vi "Main.vi"() -> ()   [LabVIEW 2015]
uses:
  Type defs/System states.ctl
  Type defs/TS UI Data.ctl
  C:/C-BOX_DoIP/Utilities/dotNET/C-BOX_DoIP/C_Box.NET_Utilities.dll
  C-BOX_DoIP/Utilities/dotNET/C-BOX_DoIP/C_Box.NET_Utilities.dll
  Type defs/Nest cluster.ctl
panel:
  in  "Nest cluster":T1={"Main messages"="", "Datamatrix"="", "Barcode"="", "Battery Voltage"="", "Scanned Hardware PN"="", "Scanned Spare PN"="", "Scanned Hardware Version"="", "Scanner Software Version"="", "Scanned Serial ID"="", "Scanned FAZIT"="", "ITAC Hardware PN"="", "ITAC Spare PN"="", "ITAC Hardware Version"="", "ITAC Software Version"="", "ITAC Serial ID"="", "ITAC FAZIT"="", "DoIP Hardware PN"="", "DoIP Spare PN"="", "DoIP Hardware Version\nDoIP Software Version"="", "DoIP Software Version"="", "DoIP Serial ID"="", "DoIP FAZIT"="", "Elapsed time"="0 seg", "Progress slider"=0.0, "System errors"=""} {"Progress slider" scale=0.1..100.0}
  in  "TestStand UI ListBar":refnum<k7>(container)
  in  "TestStand UI SequenceView":refnum<k7>(container)
  in  "Trace Enabled":refnum<k7>(container)
  in  "Sequence File Label":refnum<k7>(container) caption="Secuencia:"
  in  "Stop Button":refnum<k7>(container)
  in  "Start Button":refnum<k7>(container)
  in  "Exit Button":refnum<k7>(container)
  in  "error in (no error)":errorcluster
  in  "Reset Button":bool
  in  "Yield:":string="-"
  in  "Bad:":string="-" caption="Malas:"
  in  "Good:":string="-" caption="Buenas:"
  in  "Total:":string="-"
  in  "Info Button":bool
  in  "Settings Button":bool
  in  "TestStand UI ExecutionView Manager":refnum<k7>(container)
  in  "TestStand UI SequenceFileView Manager":refnum<k7>(container)
  in  "TestStand UI Application Manager":refnum<k7>(container)
  in  "Main message":string
  # "SCANNED DATA"
  # "ITAC DATA"
  # "DoIP DATA"
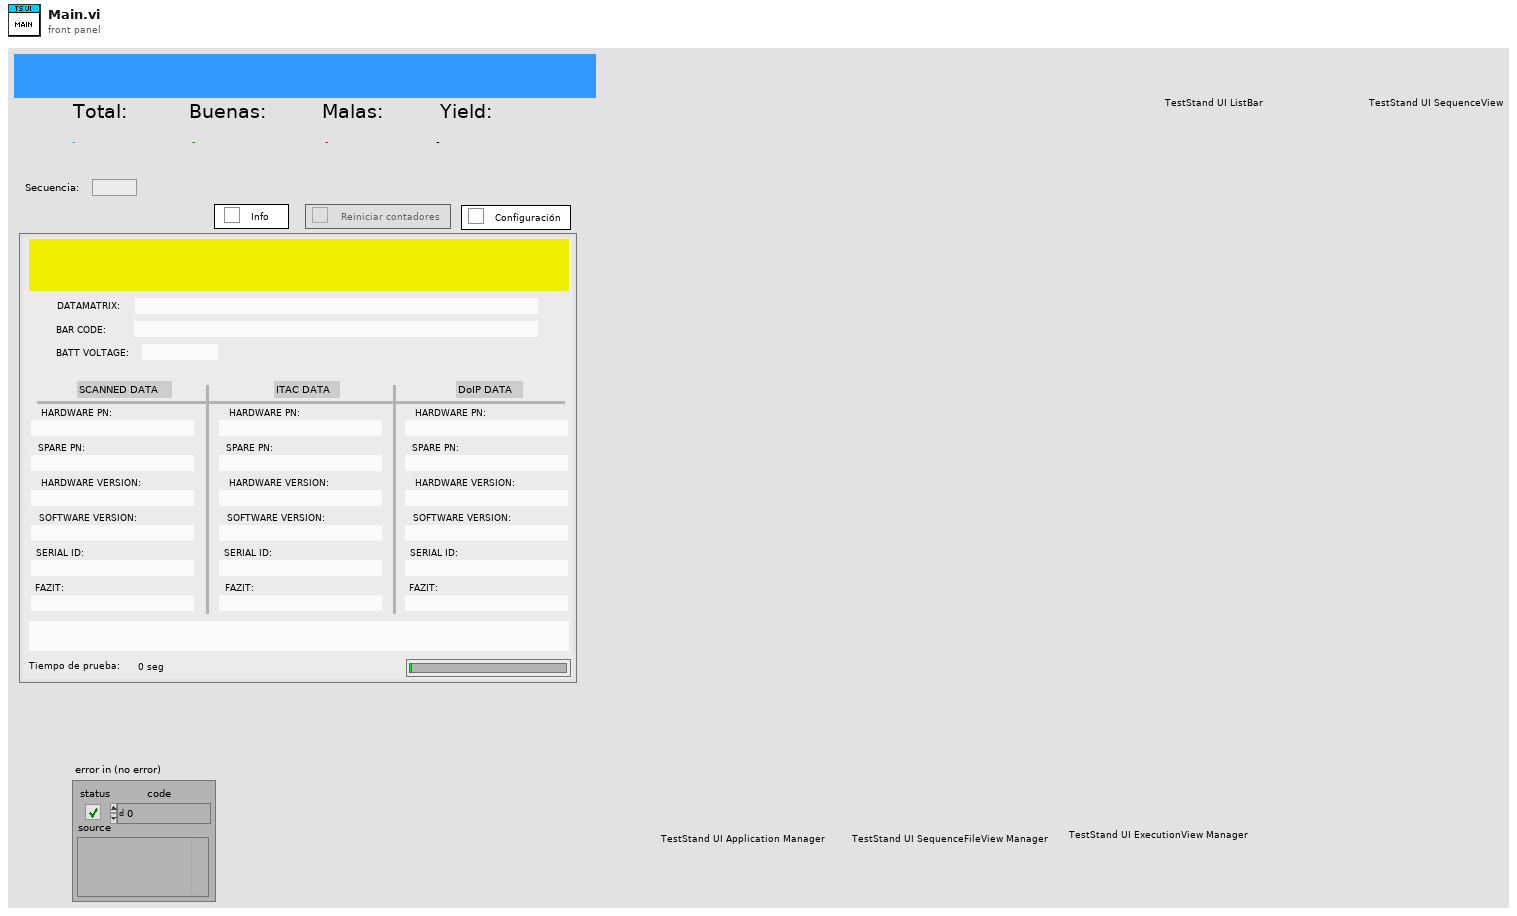
[diagram p1: front panel]
types:
  T1 = typedef "Nest cluster.ctl" = cluster{"Main messages":string, "Datamatrix":string, "Barcode":string, "Battery Voltage":string, "Scanned Hardware PN":string, "Scanned Spare PN":string, "Scanned Hardware Version":string, "Scanner Software Version":string, "Scanned Serial ID":string, "Scanned FAZIT":string, "ITAC Hardware PN":string, "ITAC Spare PN":string, "ITAC Hardware Version":string, "ITAC Software Version":string, "ITAC Serial ID":string, "ITAC FAZIT":string, "DoIP Hardware PN":string, "DoIP Spare PN":string, "DoIP Hardware Version\nDoIP Software Version":string, "DoIP Software Version":string, "DoIP Serial ID":string, "DoIP FAZIT":string, "Elapsed time":string, "Progress slider":dbl, "System errors":string}
  T2 = typedef "TS UI Data.ctl" = cluster{"Other references":cluster{"event callback refnum":refnum<k27>, "Quit Application Event":refnum<user-event>, "Change nest message bgcolor Event":refnum<user-event>, "event registration refnum":refnum<event-registration>, "Top Level VI":refnum<vi>, "TS.IEngine":refnum<k7>, "Nest Cluster":refnum<vi>}, "Manager controls":cluster{"TSUI.IApplicationMgr":refnum<k7>, "TSUI.ISequenceFileViewMgr":refnum<k7>, "TSUI.IExecutionViewMgr":refnum<k7>}, "Visible controls":cluster{"Start Button":refnum<k7>, "Stop Button":refnum<k7>, "Info Button":refnum<vi>, "Settings Button":refnum<vi>, "Reset Counters Button":refnum<vi>, "Exit Button":refnum<k7>, "Main message":refnum<vi>, "Part number":refnum<vi>, "Total counter":refnum<vi>, "Good counter":refnum<vi>, "Bad counter":refnum<vi>, "Yield":refnum<vi>, "Sequence File Label":refnum<k7>, "Trace Enabled":refnum<k7>, "Sequence View":refnum<k7>, "Sequence Execution":refnum<k7>}}
  T3 = typedef "System states.ctl" = enum16{"Init", "Configure connections", "Register callbacks", "Start application", "Event handler", "Error handler", "Shutdown"}
  T4 = enum32{"invalid app kind", "Development System", "Run Time System", "Student Edition", "Embedded LabVIEW", "Evaluation", "Custom"}
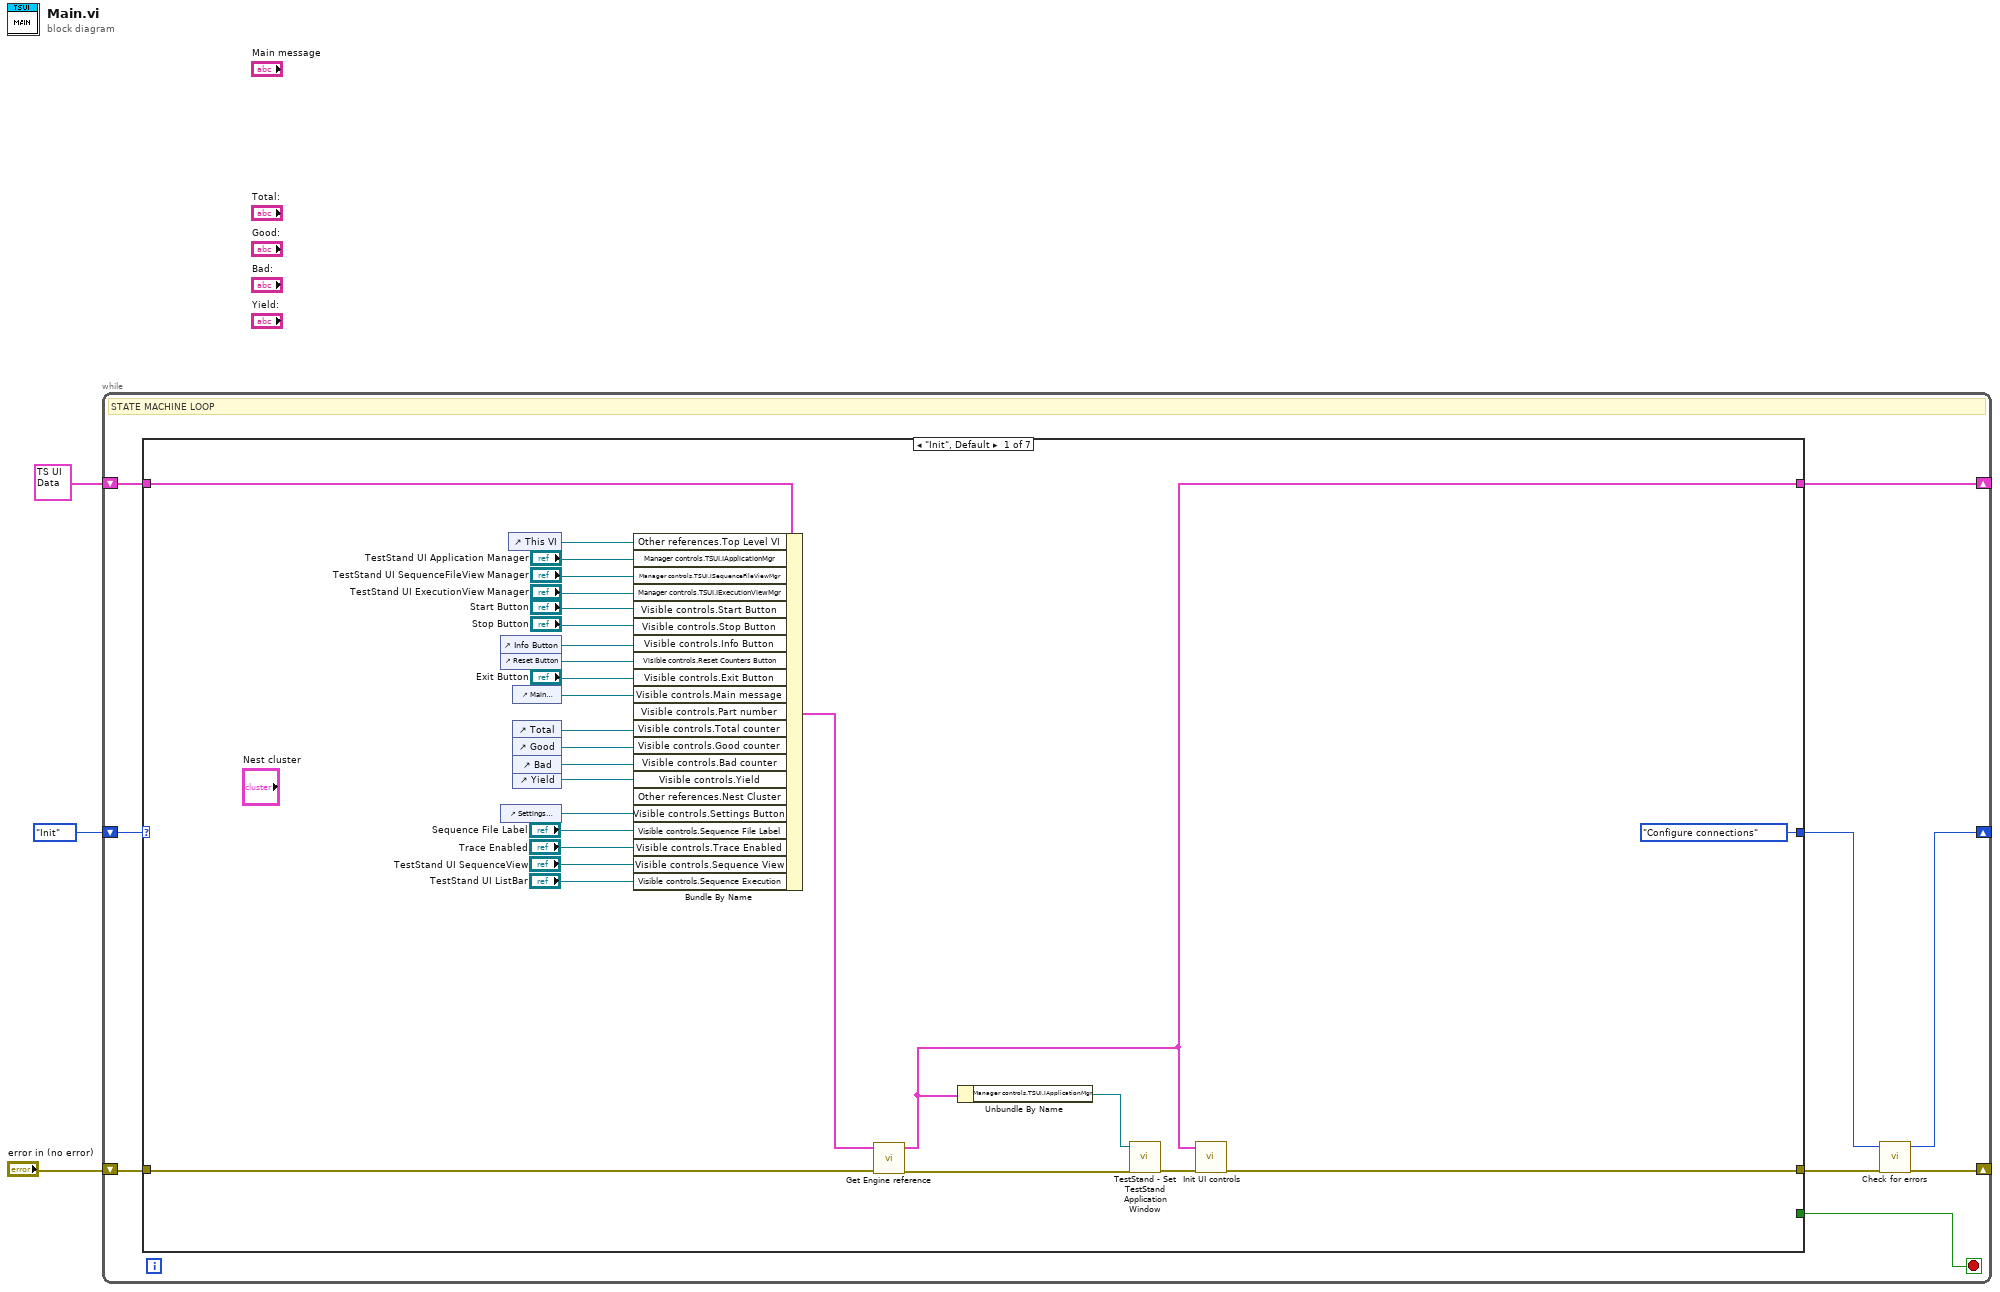
[diagram p0: block diagram]
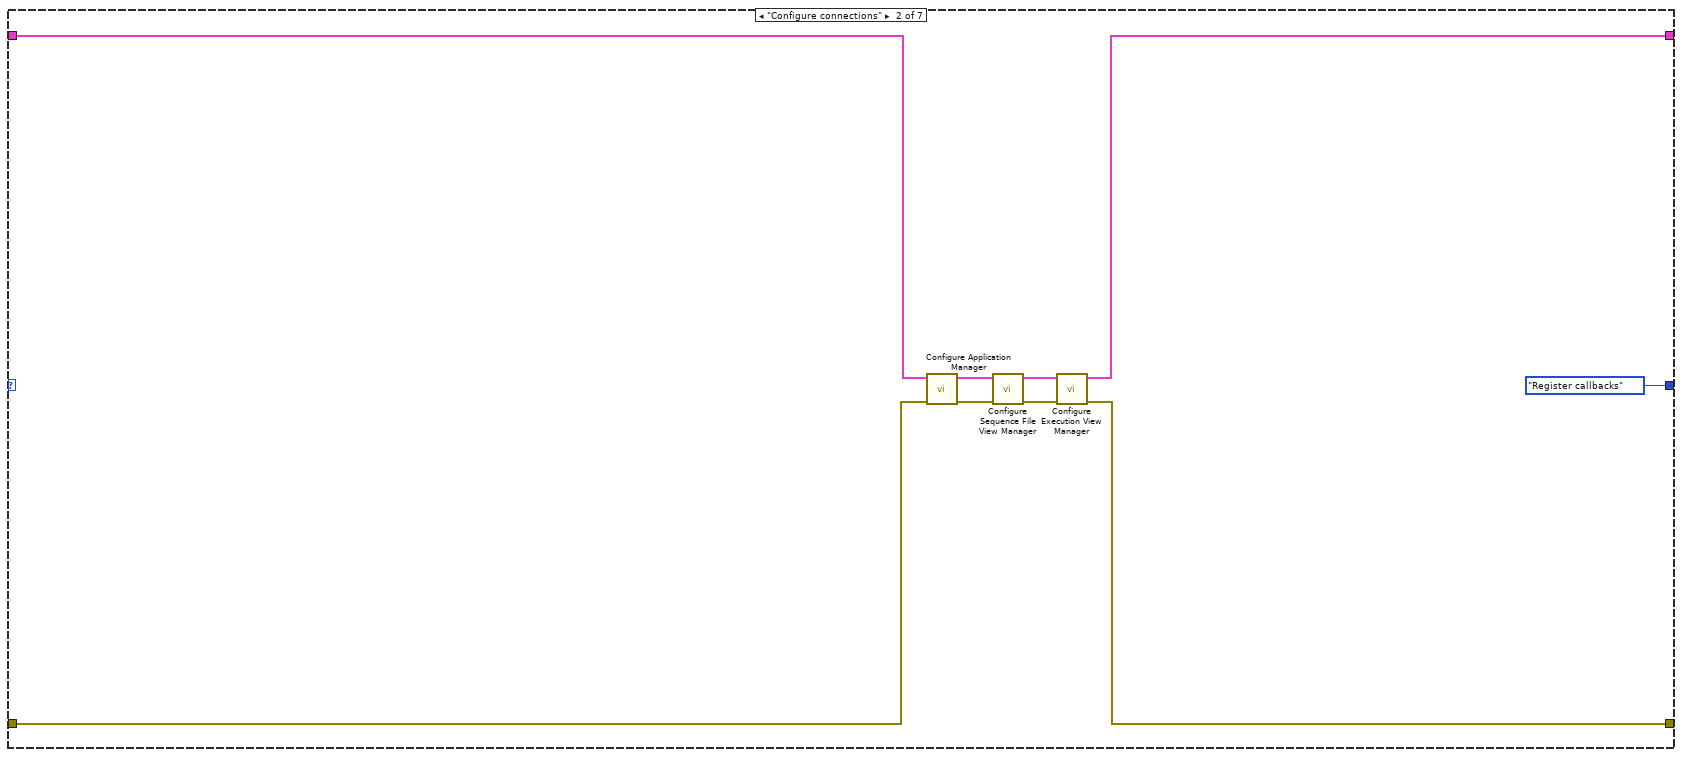
[diagram p2: hidden frame]
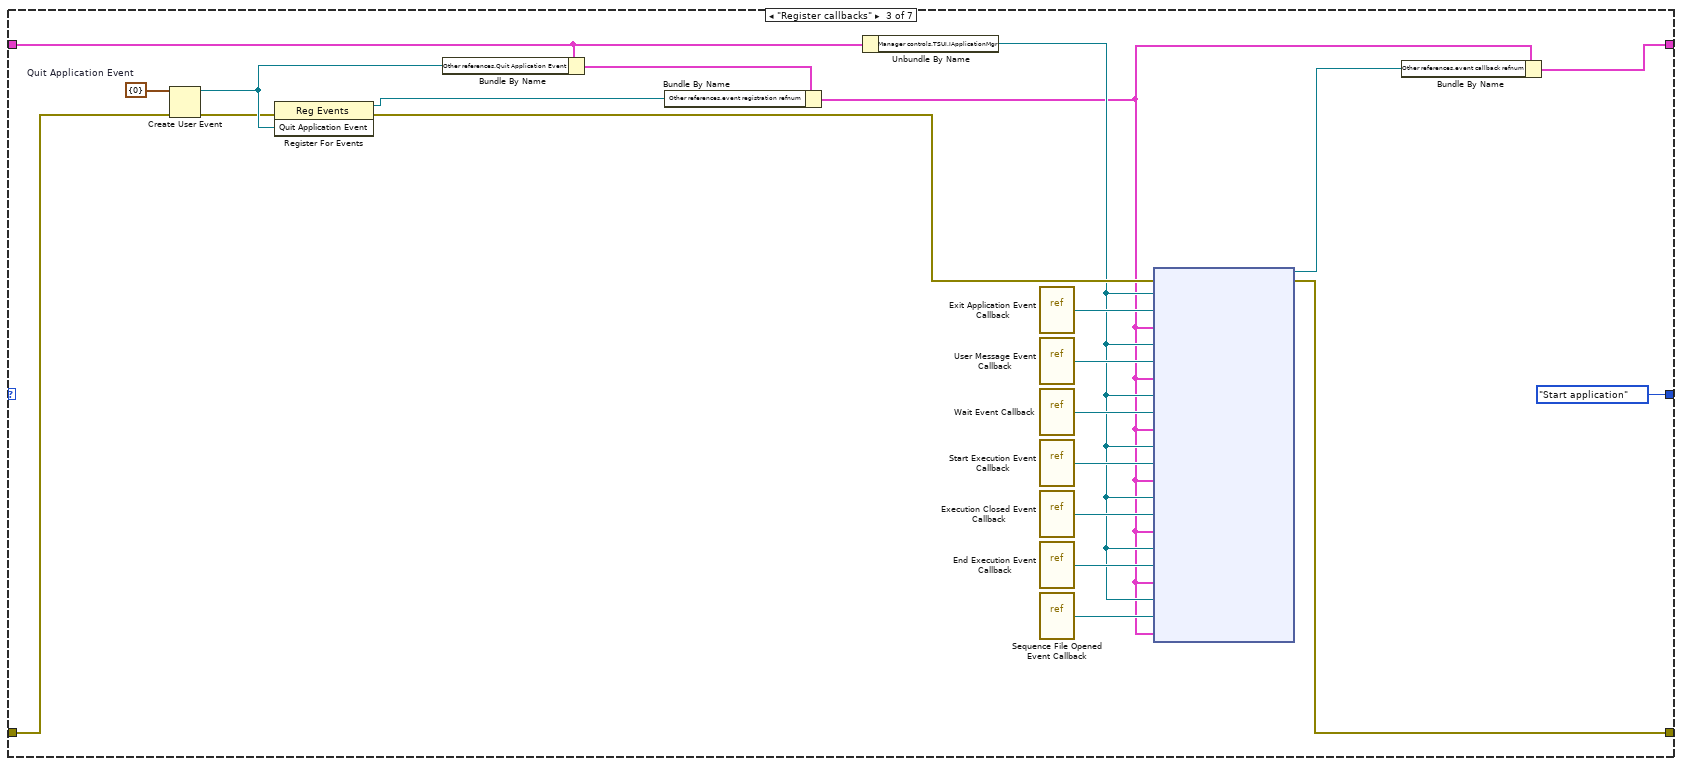
[diagram p3: hidden frame]
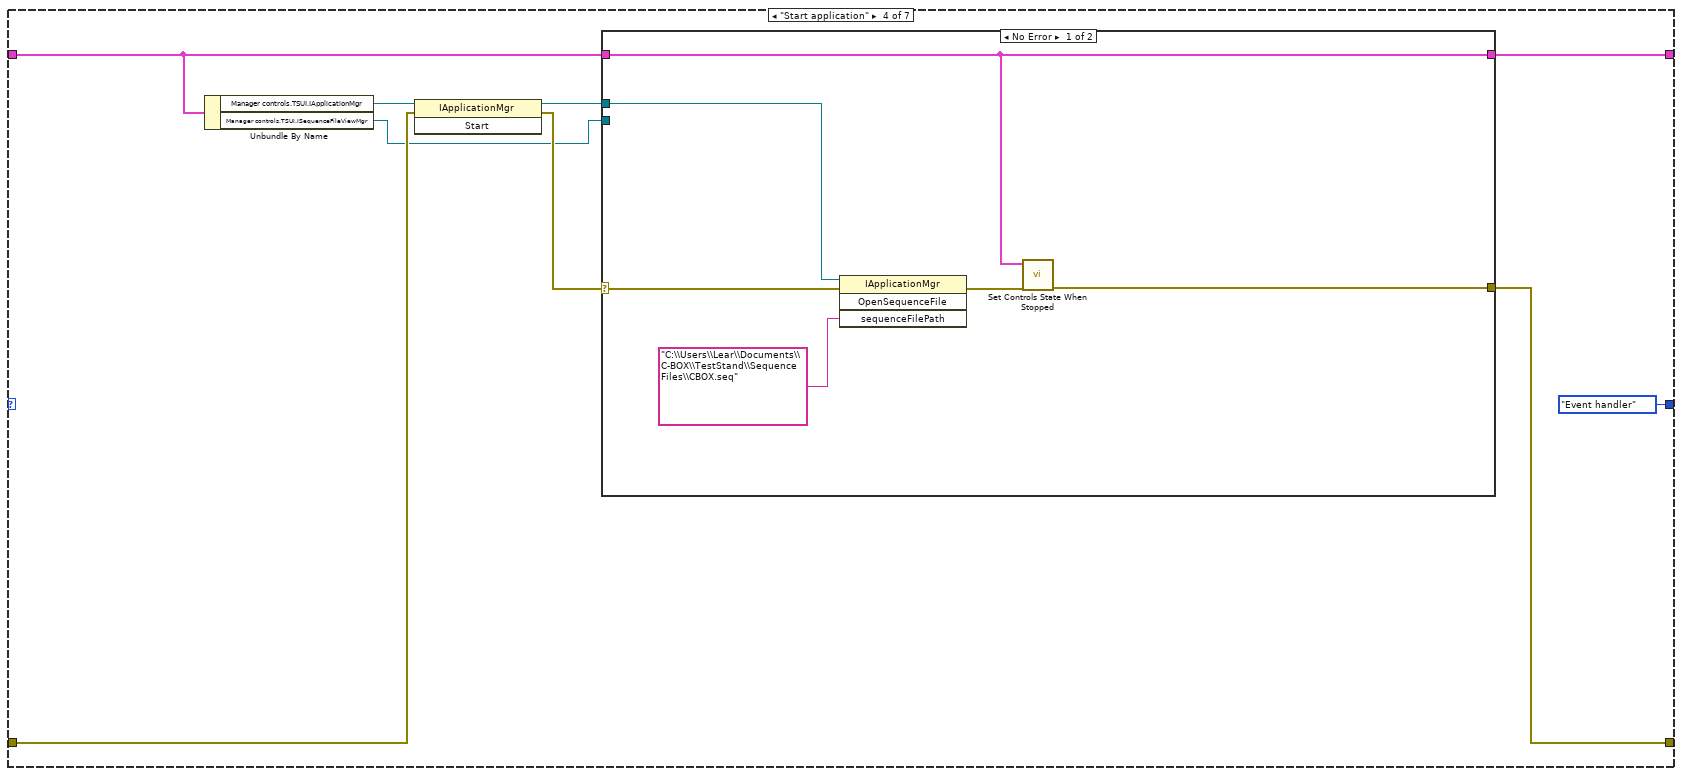
[diagram p4: hidden frame]
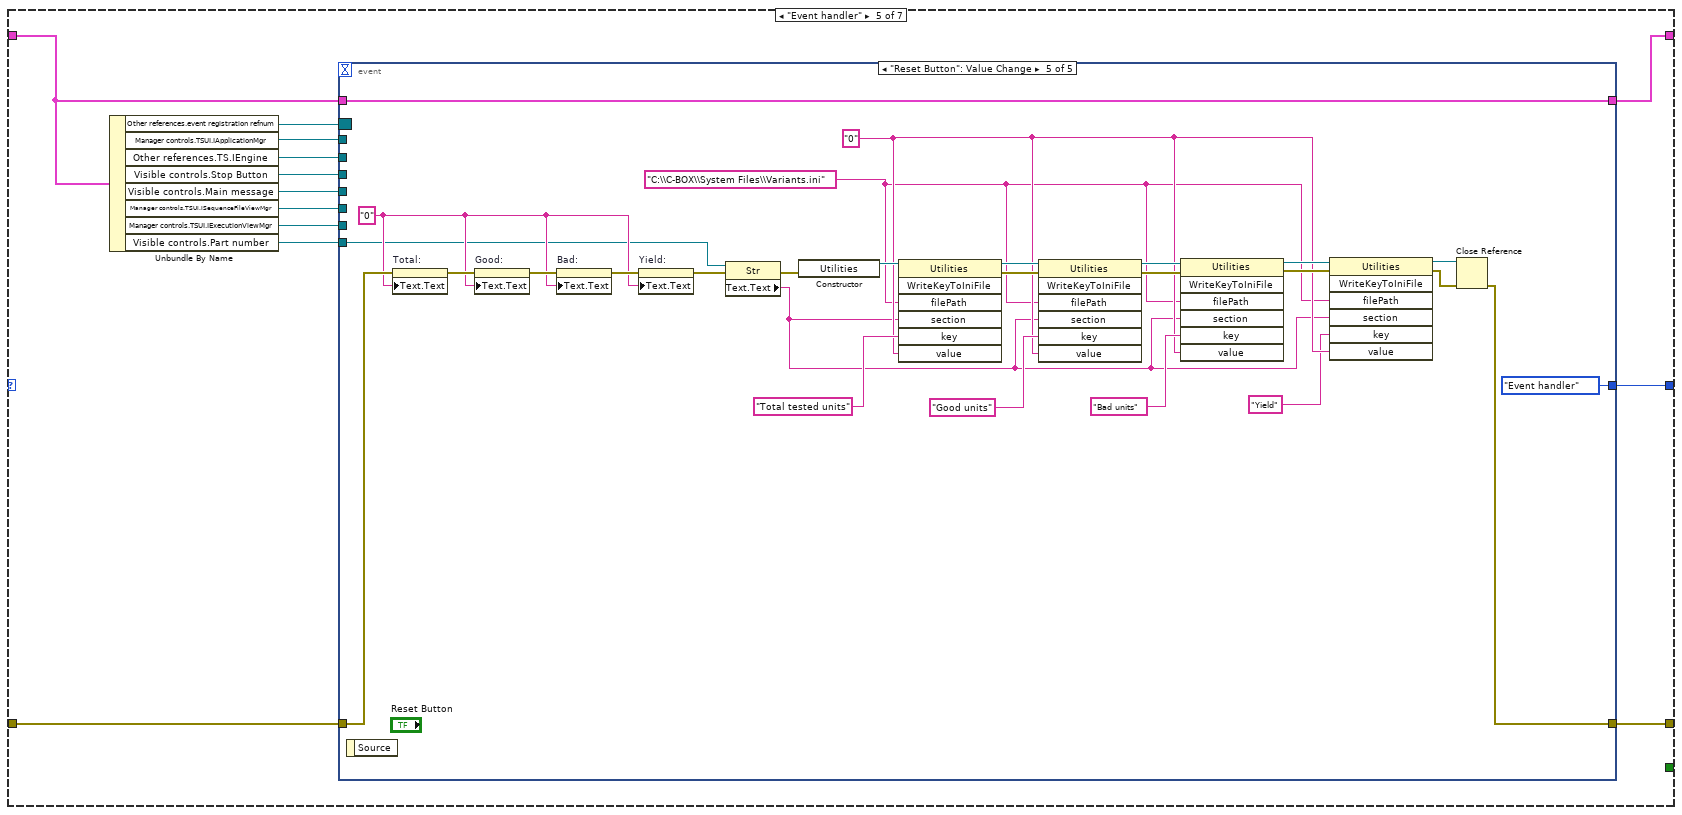
[diagram p6: hidden frame]
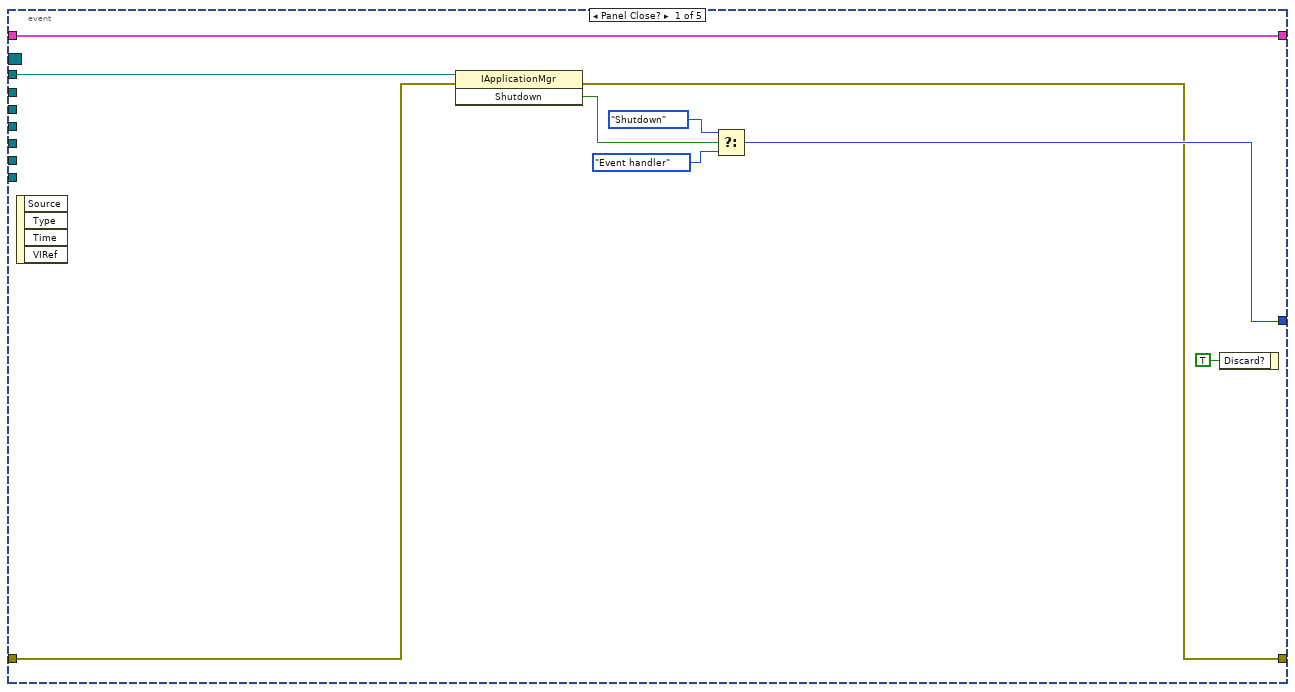
[diagram p7: hidden frame]
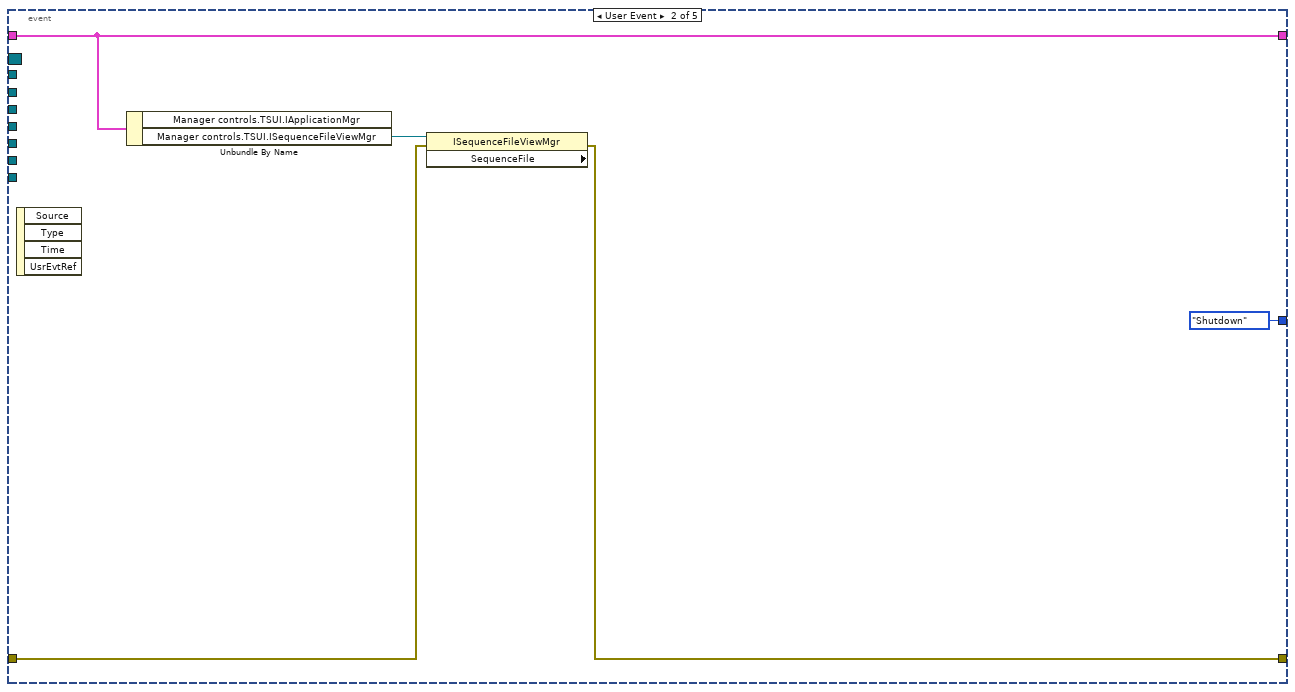
[diagram p8: hidden frame]
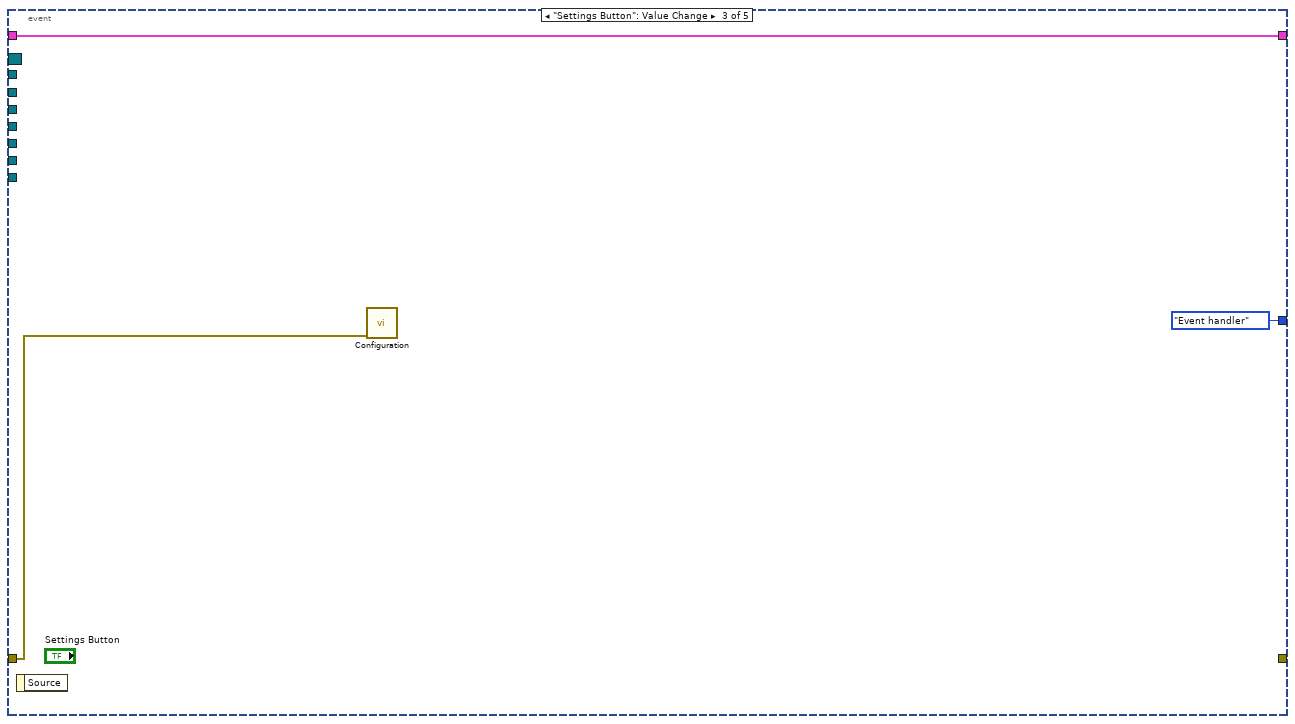
[diagram p9: hidden frame]
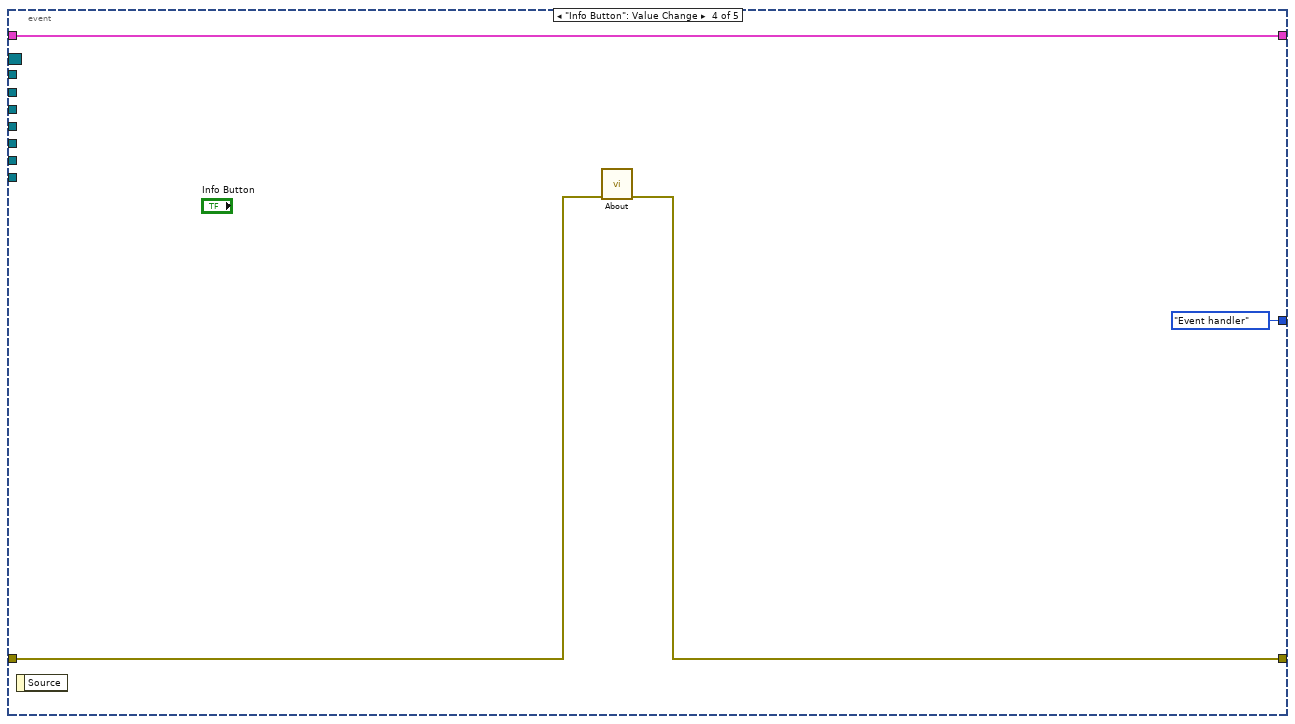
[diagram p10: hidden frame]
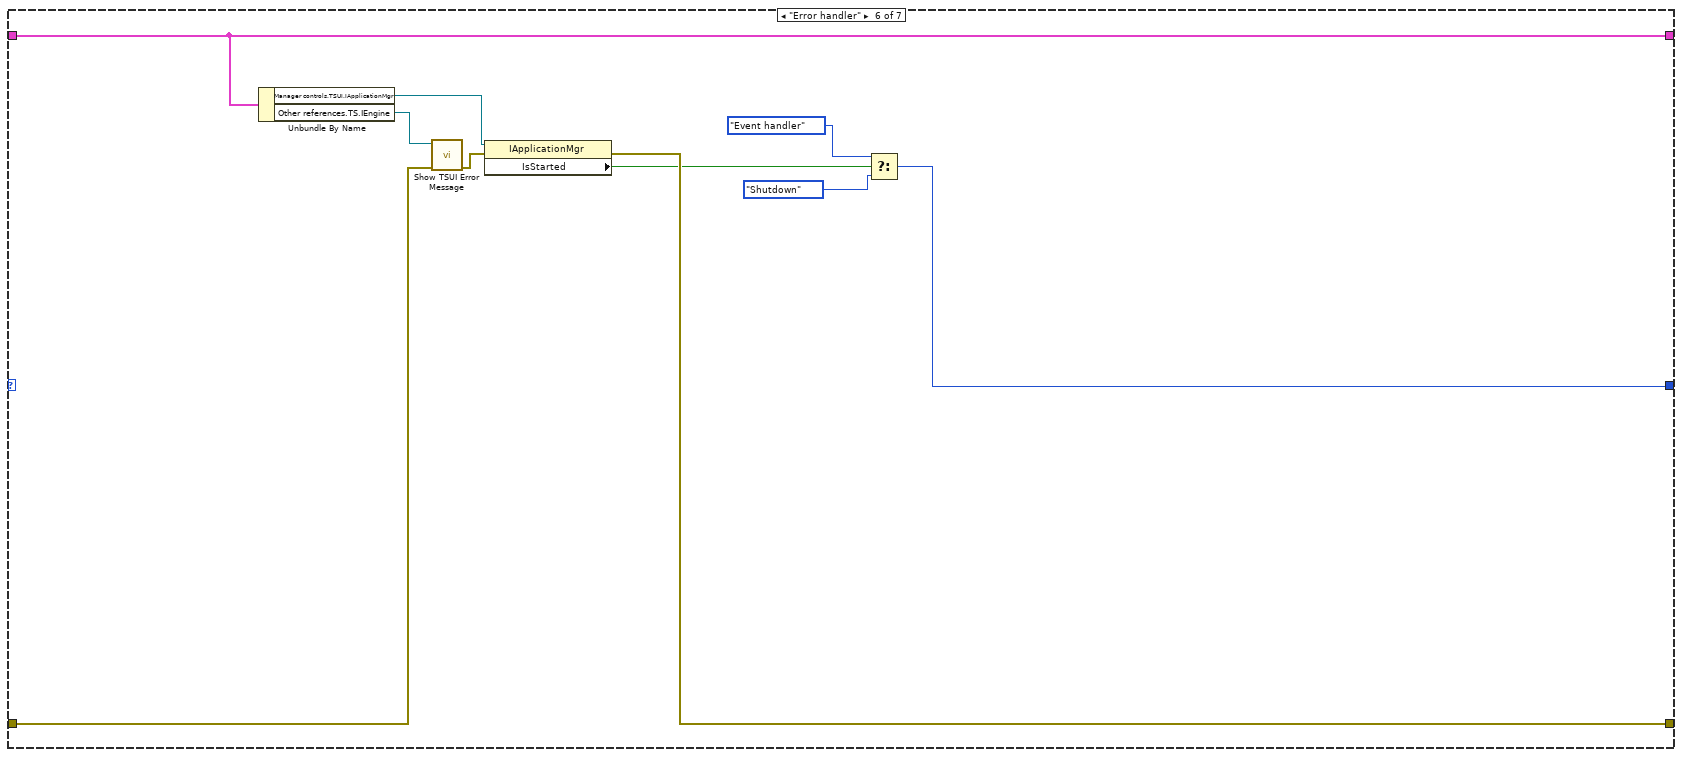
[diagram p11: hidden frame]
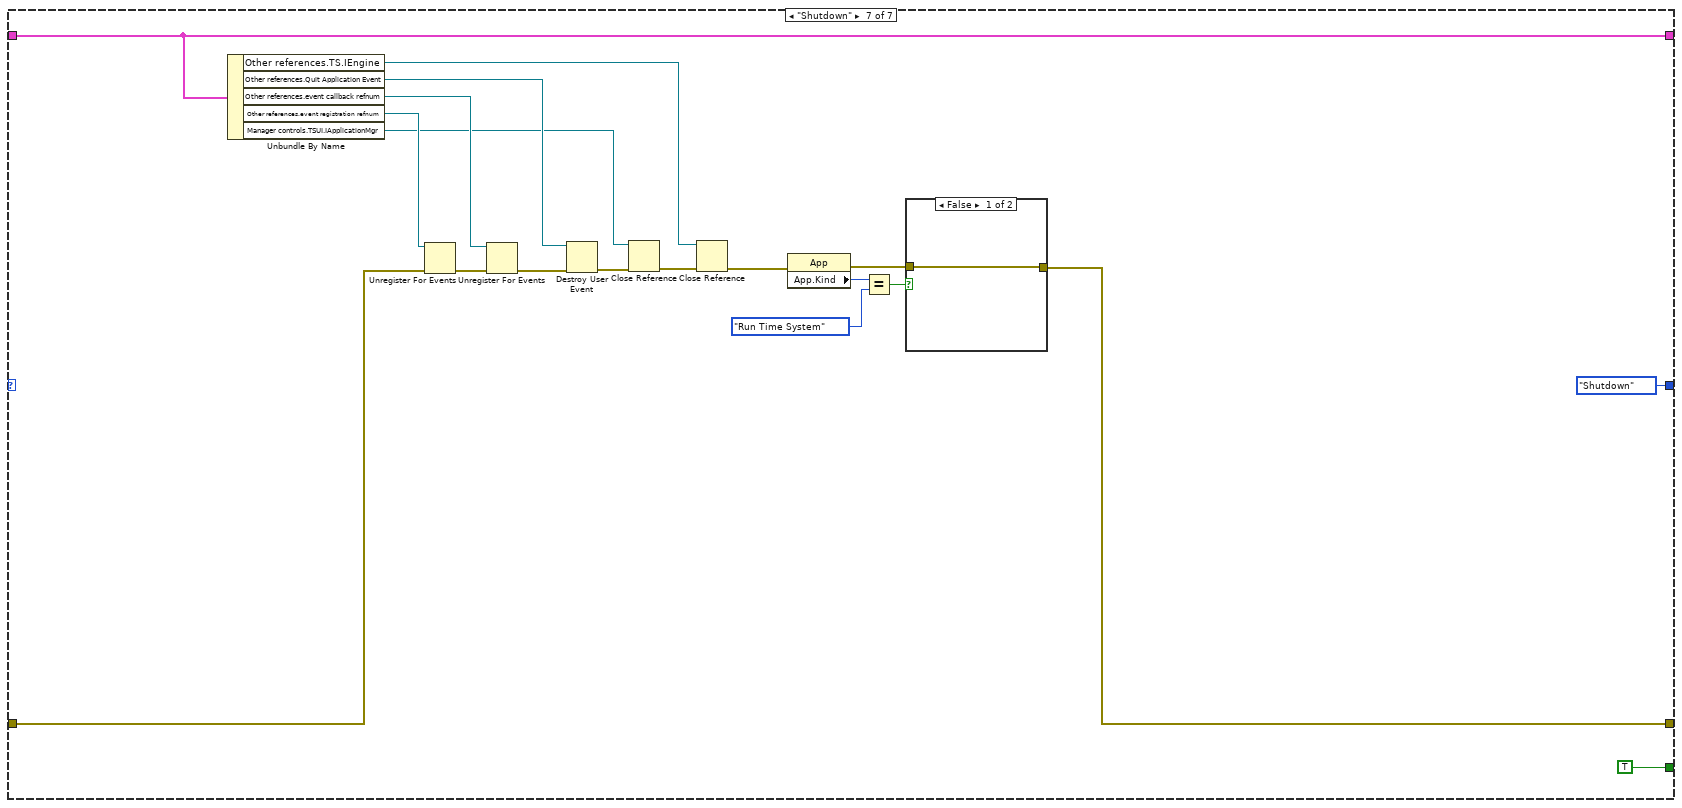
[diagram p12: hidden frame]
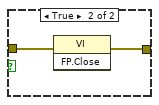
[diagram p13: hidden frame]
diagram:
  n1 = while {
    shift-right: [w7] -> _
    shift-left: "error in (no error)" -> [w9]
    shift-right: [w10] -> _
    shift-left: T2 {"Other references"={"event callback refnum"=refnum, "Quit Application Event"=refnum, "Change nest message bgcolor Event"=refnum, "event registration refnum"=refnum, "Top Level VI"=refnum, "TS.IEngine"=refnum, "Nest Cluster"=refnum}, "Manager controls"={"TSUI.IApplicationMgr"=refnum, "TSUI.ISequenceFileViewMgr"=refnum, "TSUI.IExecutionViewMgr"=refnum}, "Visible controls"={"Start Button"=refnum, "Stop Button"=refnum, "Info Button"=refnum, "Settings Button"=refnum, "Reset Counters Button"=refnum, "Exit Button"=refnum, "Main message"=refnum, "Part number"=refnum, "Total counter"=refnum, "Good counter"=refnum, "Bad counter"=refnum, "Yield"=refnum, "Sequence File Label"=refnum, "Trace Enabled"=refnum, "Sequence View"=refnum, "Sequence Execution"=refnum}} ("TS UI Data") -> [w11]
    shift-right: [w5] -> _
    shift-left: System_states."Init" ("System states") -> [w12]
    stop <- w4 stop-if-true
    # "STATE MACHINE LOOP"
    n2 = case shown="\"Init\", Default" w12 {
      tunnel: w11 -> [w42 w51 w60 w74 w94 w155 w178]
      tunnel: [w28 w45 w63 w73 w93 w155 w178] -> w10
      tunnel: [w29 w43 w62 w78 w98 w156 w165] -> w8
      tunnel: w9 -> [w32 w50 w72 w80 w99 w159 w171]
      tunnel: [System_states."Configure connections" ("System states") System_states."Register callbacks" ("System states") System_states."Start application" ("System states") System_states."Event handler" ("System states") w100 w151 System_states."Shutdown" ("System states")] -> w6
      tunnel: [_ _ _ _ _ _ TRUE] -> w4
      frame "Init", Default {
        n3 = control-ref of="Info Button"() -> (w37:refnum<vi>)
        n4 = control-ref of="Reset Button"() -> (w36:refnum<vi>)
        n5 = control-ref of="Settings Button"() -> (w18:refnum<vi>)
        n6 = control-ref of="This VI"() -> (w41:refnum<vi>)
        n7 = control-ref of="Main message"() -> (w24:refnum<vi>)
        n8 = control-ref of="Total"() -> (w22:refnum<vi>)
        n9 = control-ref of="Good"() -> (w21:refnum<vi>)
        n10 = control-ref of="Bad"() -> (w20:refnum<vi>)
        n11 = control-ref of="Yield"() -> (w19:refnum<vi>)
        n12 = Bundle By Name(cluster=w42, "Other references.Top Level VI"=w41, "Manager controls.TSUI.IApplicationMgr"="TestStand UI Application Manager", "Manager controls.TSUI.ISequenceFileViewMgr"="TestStand UI SequenceFileView Manager", "Manager controls.TSUI.IExecutionViewMgr"="TestStand UI ExecutionView Manager", "Visible controls.Start Button"="Start Button", "Visible controls.Stop Button"="Stop Button", "Visible controls.Info Button"=w37, "Visible controls.Reset Counters Button"=w36, "Visible controls.Exit Button"="Exit Button", "Visible controls.Main message"=w24, "Visible controls.Total counter"=w22, "Visible controls.Good counter"=w21, "Visible controls.Bad counter"=w20, "Visible controls.Yield"=w19, "Visible controls.Settings Button"=w18, "Visible controls.Sequence File Label"="Sequence File Label", "Visible controls.Trace Enabled"="Trace Enabled", "Visible controls.Sequence View"="TestStand UI SequenceView", "Visible controls.Sequence Execution"="TestStand UI ListBar") -> (w35:T2, "Visible controls.Part number"=w23:refnum<vi>, "Other references.Nest Cluster"=w13:refnum<vi>)
        n13 = call "Get Engine reference.vi"("error in (no error)"=w32, "TS UI Data in"=w35) -> ("error out"=w33:errorcluster, "TS UI Data out"=w28:T2)  [unwired: 8 in]
        n14 = Unbundle By Name(w28) -> ("Manager controls.TSUI.IApplicationMgr"=w34:refnum<k7>)
        n15 = call <vilib>:"TestStand - Set TestStand Application Window.vi"("error in (no error)"=w33, "Application Manager"=w34) -> ("error out"=w30:errorcluster)  [unwired: 9 in]
        n16 = call "Init UI controls.vi"("error in (no error)"=w30, "TS UI Data in"=w28) -> ("error out"=w29:errorcluster)  [unwired: 9 in]
      }
      frame "Configure connections" {
        n17 = call "Configure Application Manager.vi"("error in (no error)"=w50, "TS UI Data in"=w51) -> ("error out"=w48:errorcluster, "TS UI Data out"=w49:T2)  [unwired: 8 in]
        n18 = call "Configure Sequence File View Manager.vi"("error in (no error)"=w48, "TS UI Data in"=w49) -> ("error out"=w44:errorcluster, "TS UI Data out"=w46:T2)  [unwired: 8 in]
        n19 = call "Configure Execution View Manager.vi"("error in (no error)"=w44, "TS UI Data in"=w46) -> ("error out"=w43:errorcluster, "TS UI Data out"=w45:T2)  [unwired: 8 in]
      }
      frame "Register callbacks" {
        w57 = cluster{"Number":i32} {"Number"=0}  # Quit Application Event
        n20 = Create User Event(user event datatype=w57, error in=w72) -> (user event=w58:refnum<user-event>, error out=w52:errorcluster)
        n21 = register-events(error in=w52, w58) -> (reference out=w54:refnum<event-registration>, error out=w71:errorcluster)  [unwired: 1 in]
        n22 = Bundle By Name(cluster=w60, "Other references.Quit Application Event"=w58) -> (w56:T2)
        n23 = Bundle By Name(cluster=w56, "Other references.event registration refnum"=w54) -> (w55:T2)
        n24 = Unbundle By Name(w60) -> ("Manager controls.TSUI.IApplicationMgr"=w59:refnum<k7>)
        n25 = vi-ref "Exit Application Event Callback.vi"() -> ("vi reference"=w70:refnum<vi>)
        n26 = vi-ref "User Message Event Callback.vi"() -> ("vi reference"=w69:refnum<vi>)
        n27 = vi-ref "Wait Event Callback.vi"() -> ("vi reference"=w68:refnum<vi>)
        n28 = vi-ref "Start Execution Event Callback.vi"() -> ("vi reference"=w67:refnum<vi>)
        n29 = vi-ref "Execution Closed Event Callback.vi"() -> ("vi reference"=w66:refnum<vi>)
        n30 = vi-ref "End Execution Event Callback.vi"() -> ("vi reference"=w65:refnum<vi>)
        n31 = vi-ref "Sequence File Opened Event Callback.vi"() -> ("vi reference"=w64:refnum<vi>)
        n32 = node(w71, w59, w70, w55, w59, w69, w55, w59, w68, w55, w59, w67, w55, w59, w66, w55, w59, w65, w55, w59, w64, w55) -> (w53:refnum<k27>, w62:errorcluster)  [unwired: 1 in]
        n33 = Bundle By Name(cluster=w55, "Other references.event callback refnum"=w53) -> (w63:T2)
      }
      frame "Start application" {
        n34 = Unbundle By Name(w74) -> ("Manager controls.TSUI.IApplicationMgr"=w81:refnum<k7>, "Manager controls.TSUI.ISequenceFileViewMgr"=w75:refnum<k7>)
        n35 = invoke class="IApplicationMgr" method="Start"(reference=w81, error in=w80) -> (reference out=w76:refnum<k7>, error out=w77:errorcluster)  [unwired: 1 in, 1 out]
        n36 = case shown="No Error" w77 {
          selector: w77 -> [w84 w89]
          tunnel: [w82 w89] -> w78
          tunnel: w76 -> [w87 _]
          tunnel: w75 -> [_ _]
          tunnel: w74 -> [w85 w88]
          tunnel: [w85 w88] -> w73
          frame No Error {
            n37 = invoke class="IApplicationMgr" method="OpenSequenceFile"(reference=w87, error in=w84, "sequenceFilePath"="C:\\Users\\Lear\\Documents\\C-BOX\\TestStand\\Sequence Files\\CBOX.seq") -> (error out=w83:errorcluster)  [unwired: 1 in, 3 out]
            n38 = call "Set Controls State When Stopped.vi"("error in (no error)"=w83, "TS UI Data in"=w85) -> ("error out"=w82:errorcluster)  [unwired: 9 in]
          }
          frame Error {
          }
        }
      }
      frame "Event handler" {
        n39 = Unbundle By Name(w94) -> ("Other references.event registration refnum"=w102:refnum<event-registration>, "Manager controls.TSUI.IApplicationMgr"=w101:refnum<k7>, "Other references.TS.IEngine"=w97:refnum<k7>, "Visible controls.Stop Button"=w96:refnum<k7>, "Visible controls.Main message"=w95:refnum<vi>, "Manager controls.TSUI.ISequenceFileViewMgr"=w92:refnum<k7>, "Manager controls.TSUI.IExecutionViewMgr"=w91:refnum<k7>, "Visible controls.Part number"=w90:refnum<vi>)
        n40 = event shown="[4] \"Reset Button\": Value Change" {
          selector: w102 -> [_ _ _ _ _]
          dyn-events: _ -> [_ _ _ _ _]
          timeout: _ -> [_ _ _ _ _]
          tunnel: w101 -> [w111 _ _ _ _]
          tunnel: [w107 System_states."Shutdown" ("System states") System_states."Event handler" ("System states") System_states."Event handler" ("System states") System_states."Event handler" ("System states")] -> w100
          tunnel: w99 -> [w105 w113 w117 w122 w150]
          tunnel: [w104 w112 _ w121 w124] -> w98
          tunnel: w97 -> [_ _ _ _ _]
          tunnel: w96 -> [_ _ _ _ _]
          tunnel: w95 -> [_ _ _ _ _]
          tunnel: w94 -> [w103 w115 w118 w120 w144]
          tunnel: [w103 w115 w118 w120 w144] -> w93
          tunnel: w92 -> [_ _ _ _ _]
          tunnel: w91 -> [_ _ _ _ _]
          tunnel: w90 -> [_ _ _ _ w142]
          event Panel Close? {
            n41 = event-data() -> ()  [unwired: 1 in, 4 out]
            n42 = invoke class="IApplicationMgr" method="Shutdown"(reference=w111, error in=w105) -> (error out=w104:errorcluster, "Shutdown"=w110:bool)  [unwired: 1 in, 1 out]
            n43 = Select(t=System_states."Shutdown" ("System states"), s=w110, f=System_states."Event handler" ("System states")) -> (s? t:f=w107:T3)
            n44 = event-data("Discard?"=TRUE) -> ()  [unwired: 1 in, 1 out]
          }
          event User Event {
            n45 = event-data() -> ()  [unwired: 1 in, 4 out]
            n46 = Unbundle By Name(w115) -> ("Manager controls.TSUI.ISequenceFileViewMgr"=w114:refnum<k7>)  [unwired: 1 out]
            n47 = property class="ISequenceFileViewMgr" props=["SequenceFile"](reference=w114, error in=w113) -> (error out=w112:errorcluster)  [unwired: 2 out]
          }
          event "Settings Button": Value Change {
            n48 = event-data() -> ()  [unwired: 1 in, 1 out]
            n49 = call "Configuration.vi"("error in (no error)"=w117) -> ()  [unwired: 9 in, 2 out]
          }
          event "Info Button": Value Change {
            n50 = event-data() -> ()  [unwired: 1 in, 1 out]
            n51 = call "About.vi"("error in (no error)"=w122) -> ("error out"=w121:errorcluster)  [unwired: 10 in]
          }
          event "Reset Button": Value Change {
            w130 = "0" ("value")
            w127 = "C:\\C-BOX\\System Files\\Variants.ini" ("filePath")
            w146 = "0" ("Text.Text")
            n52 = event-data() -> ()  [unwired: 1 in, 1 out]
            n53 = property on="Total:" class="Str"(error in=w150, "Text.Text"=w146) -> (error out=w149:errorcluster)  [unwired: 1 in, 1 out]
            n54 = property on="Good:" class="Str"(error in=w149, "Text.Text"=w146) -> (error out=w148:errorcluster)  [unwired: 1 in, 1 out]
            n55 = property on="Bad:" class="Str"(error in=w148, "Text.Text"=w146) -> (error out=w147:errorcluster)  [unwired: 1 in, 1 out]
            n56 = property on="Yield:" class="Str"(error in=w147, "Text.Text"=w146) -> (error out=w141:errorcluster)  [unwired: 1 in, 1 out]
            n57 = property class="Str"(reference=w142, error in=w141) -> (error out=w140:errorcluster, "Text.Text"=w128:string)  [unwired: 1 out]
            n58 = constructor class="Utilities"(error in=w140) -> (reference out=w143:refnum<k24>)  [unwired: 2 in, 2 out]
            n59 = invoke class="Utilities" method="WriteKeyToIniFile"(reference=w143, "filePath"=w127, "section"=w128, "key"="Total tested units", "value"=w130) -> (reference out=w138:refnum<k24>, error out=w137:errorcluster)  [unwired: 2 in, 5 out]
            n60 = invoke class="Utilities" method="WriteKeyToIniFile"(reference=w138, error in=w137, "filePath"=w127, "section"=w128, "key"="Good units", "value"=w130) -> (reference out=w134:refnum<k24>, error out=w135:errorcluster)  [unwired: 1 in, 5 out]
            n61 = invoke class="Utilities" method="WriteKeyToIniFile"(reference=w134, error in=w135, "filePath"=w127, "section"=w128, "key"="Bad units", "value"=w130) -> (reference out=w132:refnum<k24>, error out=w131:errorcluster)  [unwired: 1 in, 5 out]
            n62 = invoke class="Utilities" method="WriteKeyToIniFile"(reference=w132, error in=w131, "filePath"=w127, "section"=w128, "key"="Yield", "value"=w130) -> (reference out=w126:refnum<k24>, error out=w125:errorcluster)  [unwired: 1 in, 5 out]
            n63 = Close Reference(reference=w126, error in (no error)=w125) -> (error out=w124:errorcluster)
          }
        }
      }
      frame "Error handler" {
        n64 = Unbundle By Name(w155) -> ("Manager controls.TSUI.IApplicationMgr"=w157:refnum<k7>, "Other references.TS.IEngine"=w160:refnum<k7>)
        n65 = call "Show TSUI Error Message.vi"("error in (no error)"=w159, "TS Engine Refnum in"=w160) -> ("error out"=w158:errorcluster)  [unwired: 9 in]
        n66 = property class="IApplicationMgr"(reference=w157, error in=w158) -> (error out=w156:errorcluster, "IsStarted"=w154:bool)  [unwired: 1 out]
        n67 = Select(t=System_states."Event handler" ("System states"), s=w154, f=System_states."Shutdown" ("System states")) -> (s? t:f=w151:T3)
      }
      frame "Shutdown" {
        n68 = Unbundle By Name(w178) -> ("Other references.TS.IEngine"=w161:refnum<k7>, "Other references.Quit Application Event"=w173:refnum<user-event>, "Other references.event callback refnum"=w175:refnum<k27>, "Other references.event registration refnum"=w177:refnum<event-registration>, "Manager controls.TSUI.IApplicationMgr"=w162:refnum<k7>)
        n69 = Unregister For Events(event registration refnum=w177, error in=w171) -> (error out=w176:errorcluster)
        n70 = Unregister For Events(event registration refnum=w175, error in=w176) -> (error out=w174:errorcluster)
        n71 = Destroy User Event(user event=w173, error in=w174) -> (error out=w170:errorcluster)
        n72 = Close Reference(reference=w162, error in (no error)=w170) -> (error out=w164:errorcluster)
        n73 = Close Reference(reference=w161, error in (no error)=w164) -> (error out=w163:errorcluster)
        n74 = property class="App"(error in=w163) -> (error out=w166:errorcluster, "App.Kind"=w169:T4)  [unwired: 1 in, 1 out]
        n75 = Equal?(x=w169, y=T4."Run Time System") -> (x = y?=w167:bool)
        n76 = case shown="False" w167 {
          tunnel: w166 -> [w180 w182]
          tunnel: [w180 w181] -> w165
          frame False {
          }
          frame True {
            n77 = invoke class="VI" method="FP.Close"(error in=w182) -> (error out=w181:errorcluster)  [unwired: 2 in, 2 out]
          }
        }
      }
    }
    n78 = call "Check for errors.vi"("error in (no error)"=w8, "System states in"=w6) -> ("error out"=w7:errorcluster, "System states out"=w5:T3)  [unwired: 8 in]
  }
